vi "test_ini — 2.vi"() -> ()   [LabVIEW 2016]
uses:
  <vilib>/Utility/config.llb/NI_LVConfig.lvlib
  <vilib>/Utility/config.llb/Write Key (Double).vi
  <vilib>/Utility/config.llb/Write Key (Boolean).vi
  <vilib>/Utility/config.llb/Read Key (Double).vi
  <vilib>/Utility/config.llb/Read Key (Boolean).vi
panel:
  in  "stop":bool
  in  "write":bool
  in  "Slide":dbl(slide) scale=0.0..10.0
  in  "GAS":bool
  in  "I":dbl
  in  "U":dbl
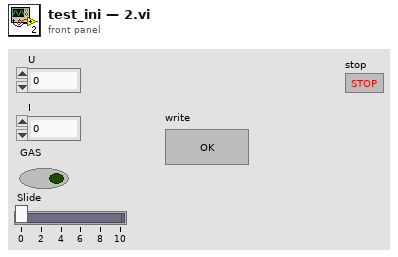
[diagram p1: front panel]
types:
  T1 = enum16{"open", "replace", "create", "open or create", "replace or create", "replace or create with confirmation"}
  T2 = typedef "NI_LVConfig.lvlib/Config Data RefNum.ctl" = refnum<k1>
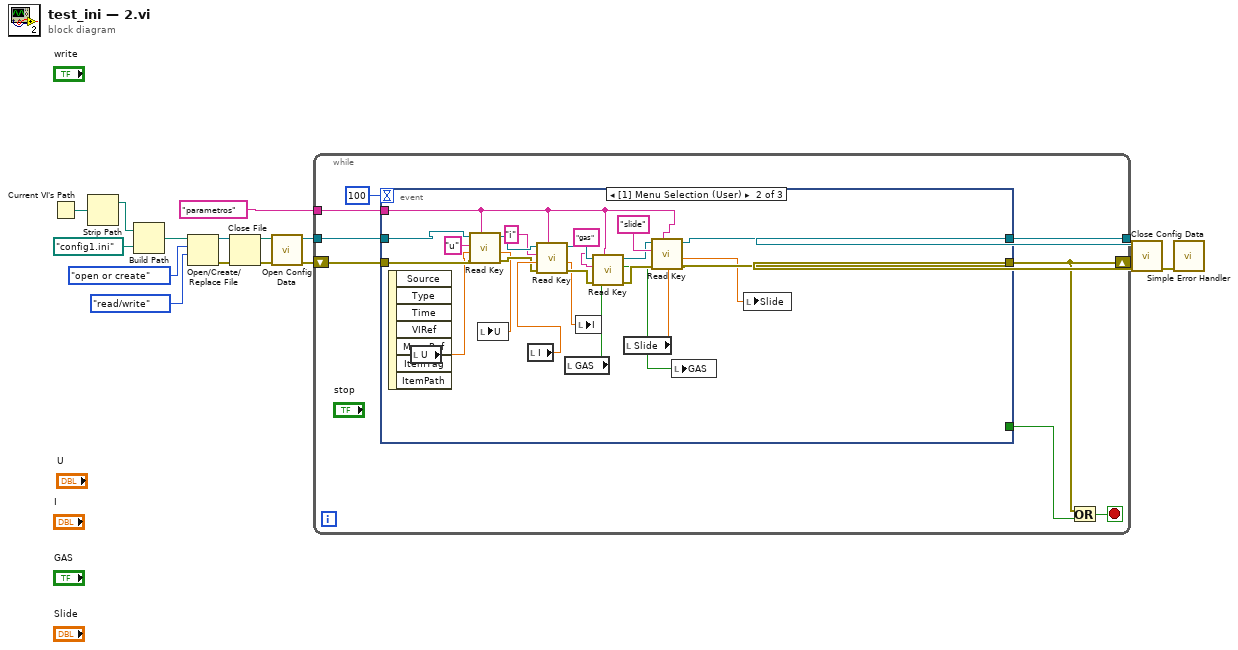
[diagram p0: block diagram]
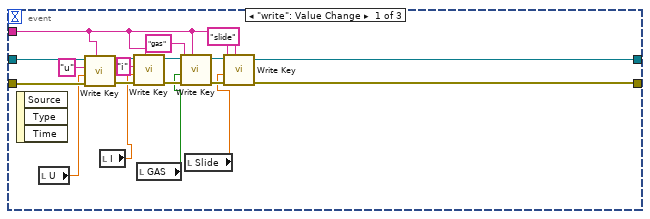
[diagram p2: hidden frame]
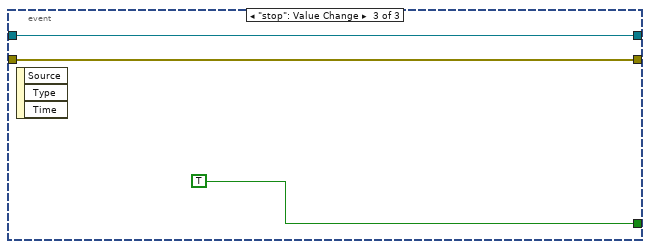
[diagram p3: hidden frame]
diagram:
  n1 = Current VI's Path() -> (path=w16:path)
  n2 = Strip Path(path=w16) -> (stripped path=w15:path)  [unwired: 1 out]
  n3 = Build Path(base path=w15, name or relative path=path "config1.ini") -> (appended path=w13:path)
  n4 = Open/Create/Replace File(file path (use dialog)=w13, operation (0:open)=T1."open or create", access (0:read/write)=enum16{"read/write", "read-only", "write-only"}."read/write") -> (refnum out=w10:refnum<file>, error out=w9:errorcluster)  [unwired: 3 in, 1 out]
  n5 = Close File(refnum=w10, error in=w9) -> (path=w8:path, error out=w1:errorcluster)
  n6 = call <vilib>:"Open Config Data.vi"("error in (no error)"=w1, "configuration file path"=w8) -> ("error out"=w6:errorcluster, "refnum"=w7:T2)  [unwired: 7 in, 1 out]
  n7 = while {
    shift-right: [w20] -> w5
    shift-left: w6 -> [w21]
    tunnel: w7 -> [w22]
    tunnel: [w19] -> w3
    tunnel: "parametros" ("section") -> [w17]
    stop <- w24 stop-if-true
    n8 = event shown="[1] Menu Selection (User)" {
      selector: _ -> [_ _ _]
      dyn-events: _ -> [_ _ _]
      timeout: 100 -> [_ _ _]
      tunnel: w22 -> [w43 w64 w69]
      tunnel: w21 -> [w42 w65 w68]
      tunnel: [w36 w61 w68] -> w20
      tunnel: [w37 w62 w69] -> w19
      tunnel: [_ _ TRUE] -> w18
      tunnel: w17 -> [w25 w55 _]
      event "write": Value Change {
        n9 = event-data() -> ()  [unwired: 1 in, 3 out]
        n10 = local read "U"() -> (w40:dbl)
        n11 = call-poly <vilib>:"Write Key.vi"("section"=w25, "error in (no error)"=w42, "value"=w40, "key"="u", "refnum"=w43) -> ("error out"=w38:errorcluster, "refnum out"=w39:T2)  [unwired: 4 in, 1 out]
        n12 = local read "I"() -> (w28:dbl)
        n13 = call-poly <vilib>:"Write Key.vi"("section"=w25, "error in (no error)"=w38, "value"=w28, "key"="i", "refnum"=w39) -> ("error out"=w32:errorcluster, "refnum out"=w33:T2)  [unwired: 4 in, 1 out]
        n14 = local read "GAS"() -> (w27:bool)
        n15 = call-poly <vilib>:"Write Key.vi"("section"=w25, "error in (no error)"=w32, "value"=w27, "key"="gas", "refnum"=w33) -> ("error out"=w35:errorcluster, "refnum out"=w34:T2)  [unwired: 4 in, 1 out]
        n16 = local read "Slide"() -> (w26:dbl)
        n17 = call-poly <vilib>:"Write Key.vi"("section"=w25, "error in (no error)"=w35, "value"=w26, "key"="slide", "refnum"=w34) -> ("error out"=w36:errorcluster, "refnum out"=w37:T2)  [unwired: 4 in, 1 out]
      }
      event Menu Selection (User) {
        n18 = event-data() -> ()  [unwired: 1 in, 7 out]
        n19 = local read "U"() -> (w63:dbl)
        n20 = call-poly <vilib>:"Read Key.vi"("section"=w55, "error in (no error)"=w65, "default value"=w63, "key"="u", "refnum"=w64) -> ("error out"=w57:errorcluster, "value"=w47:dbl, "refnum out"=w58:T2)  [unwired: 3 in, 1 out]
        n21 = local write "U"(w47) -> ()
        n22 = local read "I"() -> (w59:dbl)
        n23 = call-poly <vilib>:"Read Key.vi"("section"=w55, "error in (no error)"=w57, "default value"=w59, "key"="i", "refnum"=w58) -> ("error out"=w51:errorcluster, "value"=w46:dbl, "refnum out"=w52:T2)  [unwired: 3 in, 1 out]
        n24 = local read "GAS"() -> (w49:bool)
        n25 = local write "I"(w46) -> ()
        n26 = call-poly <vilib>:"Read Key.vi"("section"=w55, "error in (no error)"=w51, "default value"=w49, "key"="gas", "refnum"=w52) -> ("error out"=w54:errorcluster, "found?"=w45:bool, "refnum out"=w53:T2)  [unwired: 3 in, 1 out]
        n27 = local read "Slide"() -> (w48:dbl)
        n28 = call-poly <vilib>:"Read Key.vi"("section"=w55, "error in (no error)"=w54, "default value"=w48, "key"="slide", "refnum"=w53) -> ("error out"=w61:errorcluster, "value"=w44:dbl, "refnum out"=w62:T2)  [unwired: 3 in, 1 out]
        n29 = local write "GAS"(w45) -> ()
        n30 = local write "Slide"(w44) -> ()
      }
      event "stop": Value Change {
        n31 = event-data() -> ()  [unwired: 1 in, 3 out]
      }
    }
    n32 = Or(x=w20, y=w18) -> (x .or. y?=w24:bool)
  }
  n33 = call <vilib>:"Close Config Data.vi"("error in (no error)"=w5, "refnum"=w3) -> ("error out"=w4:errorcluster)  [unwired: 8 in, 1 out]
  n34 = call <vilib>:"Simple Error Handler.vi"("error in (no error)"=w4) -> ()  [unwired: 4 in, 5 out]
